vi "data to selftest.vi"(3 "byte array":u8[](array[numeric])) -> (1 "selftest":T1)   [LabVIEW 2013]
uses:
  selftest_data.ctl
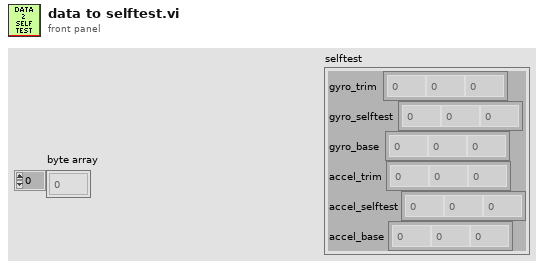
[diagram p1: front panel]
types:
  T1 = typedef "selftest_data.ctl" = cluster{"gyro_trim":u8[], "gyro_selftest":i16[], "gyro_base":i16[], "accel_trim":u8[], "accel_selftest":i16[], "accel_base":i16[]}
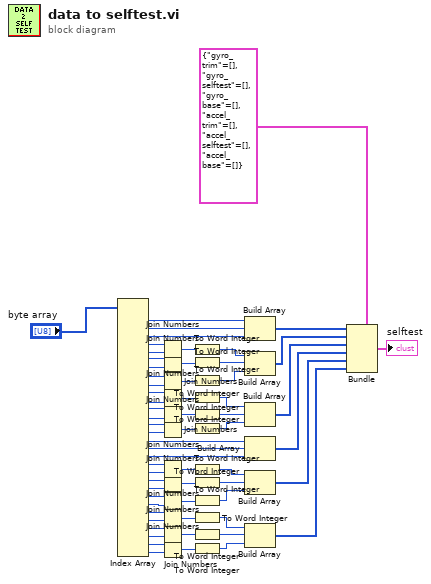
[diagram p0: block diagram]
diagram:
  n1 = Index Array(array="byte array") -> (element #1=w26:u8, element #2=w25:u8, element #3=w24:u8, element #4=w62:u8, element #5=w61:u8, element #6=w60:u8, element #7=w59:u8, element #8=w58:u8, element #9=w57:u8, element #10=w56:u8, element #11=w55:u8, element #12=w54:u8, element #13=w53:u8, element #14=w52:u8, element #15=w51:u8, element #16=w17:u8, element #17=w16:u8, element #18=w15:u8, element #19=w38:u8, element #20=w37:u8, element #21=w36:u8, element #22=w35:u8, element #23=w34:u8, element #24=w33:u8, element #25=w32:u8, element #26=w31:u8, element #27=w30:u8, element #28=w29:u8, element #29=w28:u8, element #30=w27:u8)  [unwired: 30 in]
  n2 = Join Numbers(hi=w62, lo=w61) -> ((hi.lo)=w50:u16)
  n3 = Join Numbers(hi=w60, lo=w59) -> ((hi.lo)=w49:u16)
  n4 = Join Numbers(hi=w58, lo=w57) -> ((hi.lo)=w48:u16)
  n5 = Join Numbers(hi=w56, lo=w55) -> ((hi.lo)=w47:u16)
  n6 = Join Numbers(hi=w54, lo=w53) -> ((hi.lo)=w46:u16)
  n7 = Join Numbers(hi=w52, lo=w51) -> ((hi.lo)=w45:u16)
  n8 = Join Numbers(hi=w38, lo=w37) -> ((hi.lo)=w39:u16)
  n9 = Join Numbers(hi=w36, lo=w35) -> ((hi.lo)=w40:u16)
  n10 = Join Numbers(hi=w34, lo=w33) -> ((hi.lo)=w41:u16)
  n11 = Join Numbers(hi=w32, lo=w31) -> ((hi.lo)=w42:u16)
  n12 = Join Numbers(hi=w30, lo=w29) -> ((hi.lo)=w43:u16)
  n13 = Join Numbers(hi=w28, lo=w27) -> ((hi.lo)=w44:u16)
  n14 = To Word Integer(number=w50) -> (16bit integer=w23:i16)
  n15 = To Word Integer(number=w49) -> (16bit integer=w22:i16)
  n16 = To Word Integer(number=w48) -> (16bit integer=w21:i16)
  n17 = To Word Integer(number=w47) -> (16bit integer=w19:i16)
  n18 = To Word Integer(number=w46) -> (16bit integer=w20:i16)
  n19 = To Word Integer(number=w45) -> (16bit integer=w18:i16)
  n20 = To Word Integer(number=w39) -> (16bit integer=w14:i16)
  n21 = To Word Integer(number=w40) -> (16bit integer=w13:i16)
  n22 = To Word Integer(number=w41) -> (16bit integer=w12:i16)
  n23 = To Word Integer(number=w42) -> (16bit integer=w10:i16)
  n24 = To Word Integer(number=w43) -> (16bit integer=w11:i16)
  n25 = To Word Integer(number=w44) -> (16bit integer=w9:i16)
  n26 = Build Array(w26, w25, w24) -> (w7:u8[])
  n27 = Build Array(w23, w22, w21) -> (w6:i16[])
  n28 = Build Array(w19, w20, w18) -> (w5:i16[])
  n29 = Build Array(w17, w16, w15) -> (w4:u8[])
  n30 = Build Array(w14, w13, w12) -> (w3:i16[])
  n31 = Build Array(w10, w11, w9) -> (w2:i16[])
  n32 = Bundle(cluster=T1 {"gyro_trim"=[], "gyro_selftest"=[], "gyro_base"=[], "accel_trim"=[], "accel_selftest"=[], "accel_base"=[]} ("self test data"), "gyro_trim"=w7, "gyro_selftest"=w6, "gyro_base"=w5, "accel_trim"=w4, "accel_selftest"=w3, "accel_base"=w2) -> (→"selftest":T1)
